vi "Measurement Status.vi"() -> ()   [LabVIEW 2021]
uses:
  Controls/Measurement.ctl
panel:
  out "Measurement Status":T1
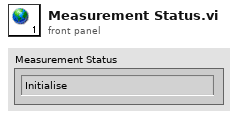
[diagram p1: front panel]
types:
  T1 = typedef "Measurement.ctl" = enum16{"Initialise", "CYL Fwd", "Wait for Delay", "CYL Rear", "Done", "Error"}
diagram:
